vi "write to sheet.vi"() -> ()   [LabVIEW 2011]
panel:
  out "String":string
  in  "Path":path
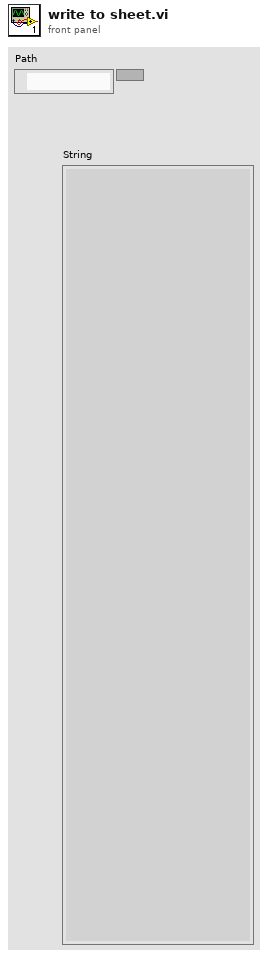
[diagram p1: front panel]
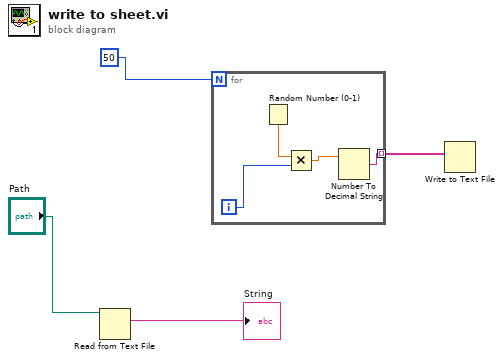
[diagram p0: block diagram]
diagram:
  n1 = Read from Text File(file (use dialog)="Path") -> (text=→"String":string)  [unwired: 3 in, 3 out]
  n2 = for {
    N: 50 -> [_]
    tunnel: [w5] -> w4 mode=indexing
    i -> [w7]
    n3 = Random Number (0-1)() -> (number: 0 to 1=w8:dbl)
    n4 = Multiply(x=w8, y=w7) -> (x*y=w6:dbl)
    n5 = Number To Decimal String(number=w6) -> (decimal integer string=w5:string)  [unwired: 1 in]
  }
  n6 = Write to Text File(text=w4) -> ()  [unwired: 3 in, 3 out]
